vi "Untitled 2.vi"   [LabVIEW 2019]
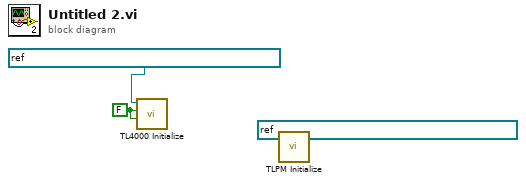
[diagram p0: block diagram]
diagram:
  w1 = FALSE ("ID Query (Do Query)")
  (unwired) refnum<visa-resource-name> "USB0::0x1313::0x807B::190927109::INSTR" ("instrument handle")
  n1 = call <instrlib>:"TL4000 Initialize.vi"("Reset Device (Reset Device)"=w1, "ID Query (Do Query)"=w1, "resource name"=refnum<visa-resource-name> "USB0::0x1313::0x804F::M00549740::INSTR" ("Diode Driver COM")) -> ()  [unwired: 7 in, 2 out]
  n2 = call <instrlib>:"TLPM Initialize.vi"() -> ()  [unwired: 10 in, 2 out]
